vi "Home.vi"(8 "error in":errorcluster, 11 "IgusMotorDrive in":refnum<class "IgusMotorDrive.lvclass">) -> (0 "error out":errorcluster, 3 "IgusMotorDrive out":refnum<class "IgusMotorDrive.lvclass">)   [LabVIEW 2016, in "IgusMotorDrive.lvclass"]
doc: "Sends the home command to the drive\n\n<b>Copyright (C) 2018 Control Software Solutions Limited. All rights reserved. </b>"
uses:
  IgusMotorDrive.lvclass
  Libraries/Modbus-Master/MB_PDU/MB_PDU_Cluster.ctl
  typedefs/Controlword--cluster.ctl
  IgusMotorDrive.lvclass/IgusMotorDrive.ctl
  Libraries/Modbus-Master/MB_Master_TCP/MB_Master_TCP.lvclass
  C:/Projekte/Lufft/CHM8K/igus Stages/igusPositioningSystem/Modules/Libraries/Modbus-Master/MB_Master/MB_Master.lvclass
  Libraries/Modbus-Master/MB Master.lvlib
panel:
  out "operation mode":u8
  out "Response":T1={"Function Code"=1, "Data"=[], "RTU_DataBytes"=0} {"Data" format="%.0x"}
  out "Command":T1={"Function Code"=1, "Data"=[], "RTU_DataBytes"=0} {"Data" format="%.0x"}
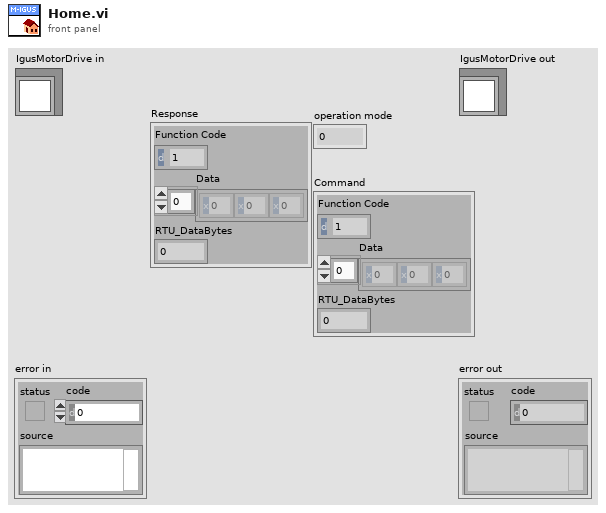
[diagram p1: front panel]
types:
  T1 = typedef "MB Master.lvlib/MB_PDU_Cluster.ctl" = cluster{"Function Code":u8, "Data":u8[], "RTU_DataBytes":i32}
  T2 = typedef "IgusMotorDrive.lvclass/Controlword--cluster.ctl" = cluster{"Switch On":bool, "Enable Voltage":bool, "Quick Stop":bool, "Enable Operation":bool, "4 MS (0: Homing Blocked/1: Homing Start) (0: No Start Signal/1: Start of Movement (0>1))":bool, "5 MS":bool, "6 MS(0:Absolute Positioning/1:Relative Positioning)":bool, "Fault Reset":bool, "8 Halt":bool, "9 MS":bool, "10 Reserved":bool, "11 Manufacturer Specific":bool, "12 Manufacturer Specific":bool, "13 Manufacturer Specific":bool, "14 Manufacturer Specific":bool, "15 Manufacturer Specific":bool}
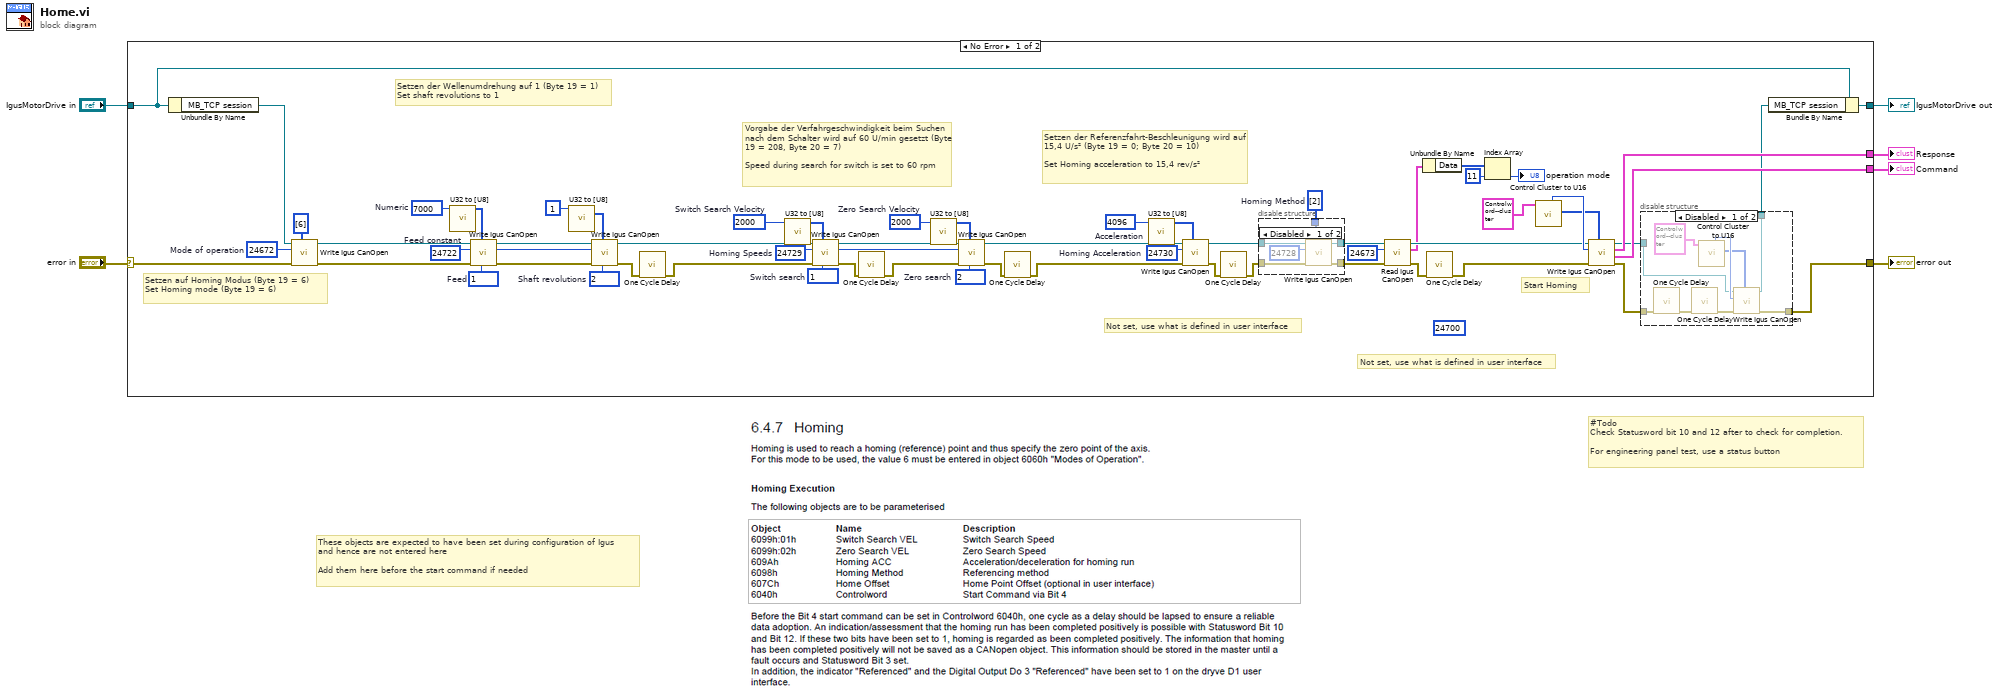
[diagram p0: block diagram]
diagram:
  # "#Todo\nCheck Statusword bit 10 and 12 after to check for completion.\n\nFor engineering panel test, use a status button"
  # "These objects are expected to have been set during configuration of Igus\nand hence are not entered here\n\nAdd them here before the start command if needed"
  n1 = case shown="No Error" "error in" {
    selector: "error in" -> [w60 w85]
    tunnel: "IgusMotorDrive in" -> [w64 w86]
    tunnel: [w65 w86] -> w4
    tunnel: [w23 w85] -> w3
    tunnel: [w54 _] -> w2
    tunnel: [w55 _] -> w1
    frame No Error {
      w19 = u32 7000  # Numeric
      w16 = u16 24722  # Feed constant
      w15 = u8 2  # Shaft revolutions
      w14 = u8 1  # Feed
      w41 = u8[] [2]  # Homing Method
      (unwired) u16 24700 ("address")
      w43 = u32 4096  # Acceleration
      w45 = u16 24730  # Homing Acceleration
      w48 = u32 2000  # Zero Search Velocity
      w50 = u32 2000  # Switch Search Velocity
      w52 = u8 2  # Zero search
      w53 = u8 1  # Switch search
      w7 = u16 24729  # Homing Speeds
      w62 = u16 24672  # Mode of operation
      # "Start Homing"
      # "Setzen der Referenzfahrt-Beschleunigung wird auf 15,4 U/s² (Byte 19 = 0; Byte 20 = 10)\n\nSet Homing acceleration to 15,4 rev/s²"
      # "Vorgabe der Verfahrgeschwindigkeit beim Suchen nach dem Schalter wird auf 60 U/min gesetzt (Byte 19 = 208, Byte 20 = 7)\n\nSpeed during search for switch is set to 60 rpm"
      # "Setzen der Wellenumdrehung auf 1 (Byte 19 = 1)\nSet shaft revolutions to 1"
      # "Setzen auf Homing Modus (Byte 19 = 6)\nSet Homing mode (Byte 19 = 6)"
      # "Not set, use what is defined in user interface"
      # "Not set, use what is defined in user interface"
      n2 = Unbundle By Name(w64) -> ("MB_TCP session"=w59:refnum<class "MB_Master_TCP.lvclass">)
      n3 = call "Write Igus CanOpen.vi"("Data [1-4]"=u8[] [6], "error in (no error)"=w60, "Address"=w62, "MB session in"=w59) -> ("error out"=w11:errorcluster, "MB session out"=w9:refnum<class "MB_Master_TCP.lvclass">)  [unwired: 4 in, 2 out]
      n4 = call "U32 to [U8].vi"("Numeric"=w19) -> ("output array"=w18:u8[])  [unwired: 10 in]
      n5 = call "Write Igus CanOpen.vi"("Sub Index"=w14, "Data [1-4]"=w18, "error in (no error)"=w11, "Address"=w16, "MB session in"=w9) -> ("error out"=w12:errorcluster, "MB session out"=w13:refnum<class "MB_Master_TCP.lvclass">)  [unwired: 3 in, 2 out]
      n6 = call "U32 to [U8].vi"("Numeric"=u32 1) -> ("output array"=w17:u8[])  [unwired: 10 in]
      n7 = call "Write Igus CanOpen.vi"("Sub Index"=w15, "Data [1-4]"=w17, "error in (no error)"=w12, "Address"=w16, "MB session in"=w13) -> ("error out"=w10:errorcluster, "MB session out"=w8:refnum<class "MB_Master_TCP.lvclass">)  [unwired: 3 in, 2 out]
      n8 = call "One Cycle Delay.vi"("error in"=w10) -> ("error out"=w40:errorcluster)  [unwired: 10 in]
      n9 = call "U32 to [U8].vi"("Numeric"=w50) -> ("output array"=w49:u8[])  [unwired: 10 in]
      n10 = call "Write Igus CanOpen.vi"("Sub Index"=w53, "Data [1-4]"=w49, "error in (no error)"=w40, "Address"=w7, "MB session in"=w8) -> ("error out"=w39:errorcluster, "MB session out"=w51:refnum<class "MB_Master_TCP.lvclass">)  [unwired: 3 in, 2 out]
      n11 = call "One Cycle Delay.vi"("error in"=w39) -> ("error out"=w38:errorcluster)  [unwired: 10 in]
      n12 = call "U32 to [U8].vi"("Numeric"=w48) -> ("output array"=w47:u8[])  [unwired: 10 in]
      n13 = call "Write Igus CanOpen.vi"("Sub Index"=w52, "Data [1-4]"=w47, "error in (no error)"=w38, "Address"=w7, "MB session in"=w51) -> ("error out"=w37:errorcluster, "MB session out"=w46:refnum<class "MB_Master_TCP.lvclass">)  [unwired: 3 in, 2 out]
      n14 = call "One Cycle Delay.vi"("error in"=w37) -> ("error out"=w36:errorcluster)  [unwired: 10 in]
      n15 = call "U32 to [U8].vi"("Numeric"=w43) -> ("output array"=w44:u8[])  [unwired: 10 in]
      n16 = call "Write Igus CanOpen.vi"("Data [1-4]"=w44, "error in (no error)"=w36, "Address"=w45, "MB session in"=w46) -> ("error out"=w35:errorcluster, "MB session out"=w42:refnum<class "MB_Master_TCP.lvclass">)  [unwired: 4 in, 2 out]
      n17 = call "One Cycle Delay.vi"("error in"=w35) -> ("error out"=w34:errorcluster)  [unwired: 10 in]
      n18 = disable-structure shown="Disabled" {
        disable-tunnel: w42 -> [w70 w72]
        disable-tunnel: w41 -> [w69 _]
        disable-tunnel: w34 -> [w68 w73]
        disable-tunnel: [w67 w73] -> w33
        disable-tunnel: [w66 w72] -> w31
        frame Disabled {
          n19 = call "Write Igus CanOpen.vi"("Data [1-4]"=w69, "error in (no error)"=w68, "Address"=u16 24728 ("address"), "MB session in"=w70) -> ("error out"=w67:errorcluster, "MB session out"=w66:refnum<class "MB_Master_TCP.lvclass">)  [unwired: 4 in, 2 out]
        }
        frame Enabled {
        }
      }
      n20 = call "Read Igus CanOpen.vi"("error in (no error)"=w33, "Address"=u16 24673 ("address"), "MB session in"=w31) -> ("error out"=w32:errorcluster, "Response"=w28:T1, "MB session out"=w30:refnum<class "MB_Master_TCP.lvclass">)  [unwired: 5 in, 1 out]
      n21 = Unbundle By Name(w28) -> ("Data"=w27:u8[])
      n22 = call "One Cycle Delay.vi"("error in"=w32) -> ("error out"=w56:errorcluster)  [unwired: 10 in]
      n23 = Index Array(array=w27, index=11) -> (element=→"operation mode":u8)
      n24 = call "Control Cluster to U16.vi"("Controlword"=T2 {"Switch On"=TRUE, "Enable Voltage"=TRUE, "Quick Stop"=TRUE, "Enable Operation"=TRUE, "4 MS (0: Homing Blocked/1: Homing Start) (0: No Start Signal/1: Start of Movement (0>1))"=TRUE, "5 MS"=FALSE, "6 MS(0:Absolute Positioning/1:Relative Positioning)"=FALSE, "Fault Reset"=FALSE, "8 Halt"=FALSE, "9 MS"=FALSE, "10 Reserved"=FALSE, "11 Manufacturer Specific"=FALSE, "12 Manufacturer Specific"=FALSE, "13 Manufacturer Specific"=FALSE, "14 Manufacturer Specific"=FALSE, "15 Manufacturer Specific"=FALSE}) -> ("Control word Data"=w57:u8[], "address"=w58:u16)  [unwired: 8 in, 1 out]
      n25 = call "Write Igus CanOpen.vi"("Data [1-4]"=w57, "error in (no error)"=w56, "Address"=w58, "MB session in"=w30) -> ("error out"=w24:errorcluster, "Command"=w54:T1, "Response"=w55:T1, "MB session out"=w22:refnum<class "MB_Master_TCP.lvclass">)  [unwired: 4 in]
      n26 = disable-structure shown="Disabled" {
        disable-tunnel: w24 -> [w82 w84]
        disable-tunnel: [w81 w84] -> w23
        disable-tunnel: w22 -> [w78 w83]
        disable-tunnel: [w77 w83] -> w21
        frame Disabled {
          n27 = call "One Cycle Delay.vi"("error in"=w82) -> ("error out"=w74:errorcluster)  [unwired: 10 in]
          n28 = call "One Cycle Delay.vi"("error in"=w74) -> ("error out"=w75:errorcluster)  [unwired: 10 in]
          n29 = call "Control Cluster to U16.vi"("Controlword"=T2 {"Switch On"=TRUE, "Enable Voltage"=TRUE, "Quick Stop"=TRUE, "Enable Operation"=TRUE, "4 MS (0: Homing Blocked/1: Homing Start) (0: No Start Signal/1: Start of Movement (0>1))"=FALSE, "5 MS"=FALSE, "6 MS(0:Absolute Positioning/1:Relative Positioning)"=FALSE, "Fault Reset"=FALSE, "8 Halt"=FALSE, "9 MS"=FALSE, "10 Reserved"=FALSE, "11 Manufacturer Specific"=FALSE, "12 Manufacturer Specific"=FALSE, "13 Manufacturer Specific"=FALSE, "14 Manufacturer Specific"=FALSE, "15 Manufacturer Specific"=FALSE}) -> ("Control word Data"=w76:u8[], "address"=w79:u16)  [unwired: 8 in, 1 out]
          n30 = call "Write Igus CanOpen.vi"("Data [1-4]"=w76, "error in (no error)"=w75, "Address"=w79, "MB session in"=w78) -> ("error out"=w81:errorcluster, "MB session out"=w77:refnum<class "MB_Master_TCP.lvclass">)  [unwired: 4 in, 2 out]
        }
        frame Enabled {
        }
      }
      n31 = Bundle By Name(cluster=w64, "MB_TCP session"=w21) -> (w65:refnum<class "IgusMotorDrive.lvclass">)
    }
    frame Error {
    }
  }
  "error out" <- w3
  "IgusMotorDrive out" <- w4
  "Command" <- w2
  "Response" <- w1
